vi "Checkout Master File.vi"(8 "error in":errorcluster, 10 "File Index":i32, 11 "Peer Review in":refnum<class "Peer Review.lvclass">) -> (0 "error out":errorcluster, 3 "Peer Review out":refnum<class "Peer Review.lvclass">)   [LabVIEW 2020, in "Peer Review.lvclass"]
uses:
  Peer Review.lvclass
  Peer Review.lvclass/Peer Review.ctl
  TypeDefs/File State.ctl
  <vilib>/security/Message Digest/API/Instances/File/SHA-256 File Checksum.vi
  <vilib>/security/Message Digest/API/NI_Message Digest API.lvlib
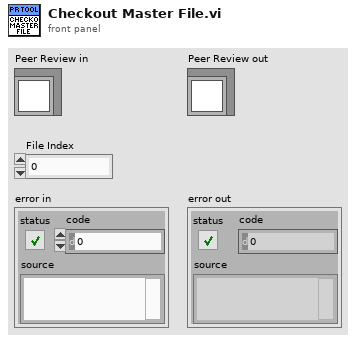
[diagram p1: front panel]
types:
  T1 = typedef "Peer Review.lvclass/File State.ctl" = enum16{"Interrogation Needed", "Modified", "Deleted", "Added", "Matches Previous", "No Changes", "Moved"}
  T2 = typedef "Peer Review.lvclass/File Info.ctl" = cluster{"File ID":i32, "Commit ID":i32, "Reviewed Hash":string, "Relative Path":string, "File Path":path, "File Checksum":string, "State":T1, "FP Changes":i32, "BD Changes":i32, "FP Bounds Error":dbl, "BD Bounds Error":dbl, "Lines Added":i32, "Lines Removed":i32, "Analysis Passes":i32, "Analysis Fails":i32, "Attribute Changes":i32, "Reentrancy State":string, "Cyclomatic Complexity":i32, "Node Count":i32, "Revision Number":u32, "LabVIEW Version":string, "Description":string, "Master Path":path, "Master Checksum":string, "VI Type":T3, "LabVIEW File":bool, "Review Complete":bool, "File Ref":refnum<vi>}
  T3 = typedef "Peer Review.lvclass/VI Type.ctl" = enum32{"invalid VI type", "Standard VI", "Control VI", "Global VI", "Polymorphic VI", "Configuration VI", "SubSystem", "Facade VI", "Method VI", "Statechart Diagram VI"}
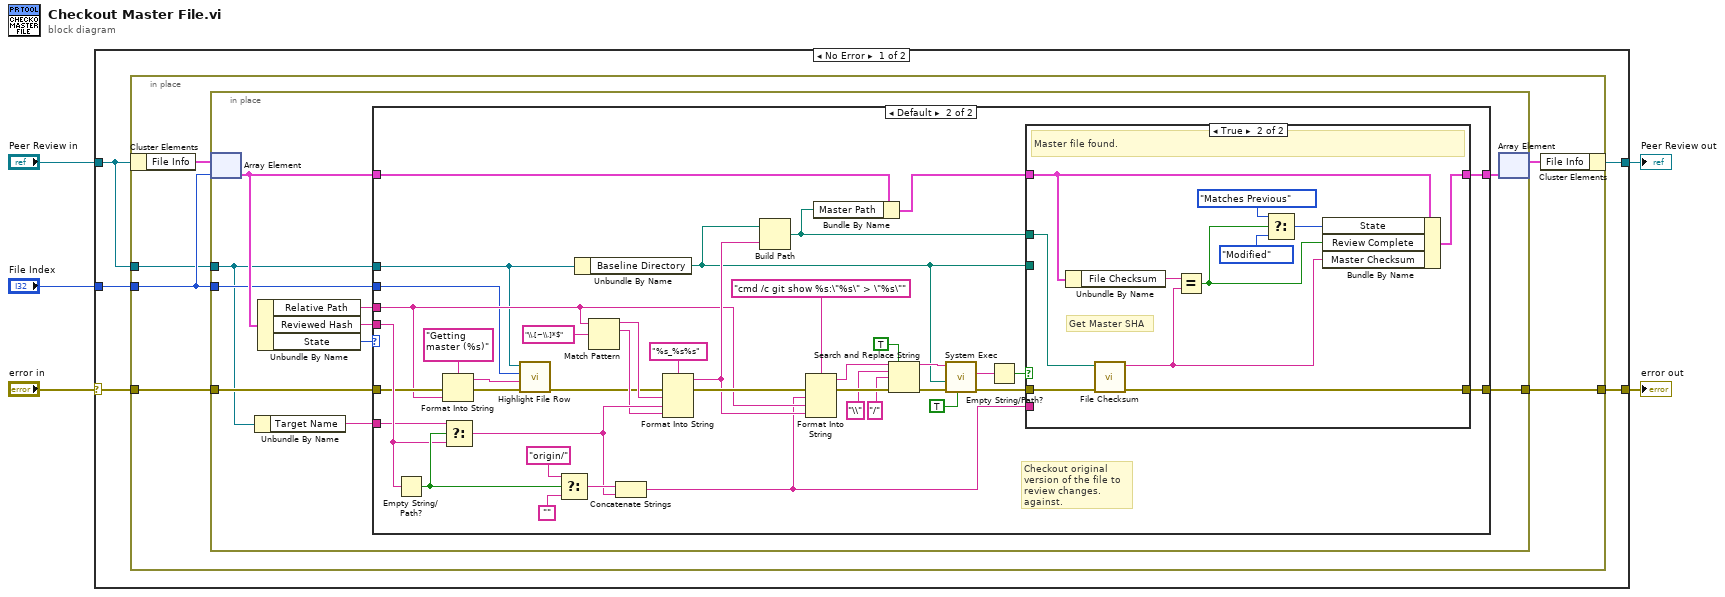
[diagram p0: block diagram]
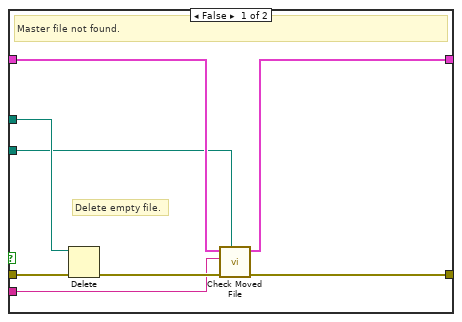
[diagram p3: hidden frame]
diagram:
  n1 = case shown="No Error" "error in" {
    selector: "error in" -> [w10 w89]
    tunnel: [w9 w89] -> w4
    tunnel: "Peer Review in" -> [w6 w88]
    tunnel: "File Index" -> [w8 _]
    tunnel: [w7 w88] -> w1
    frame No Error {
      n2 = in-place {
        in-place-border: w10 -> [w16]
        in-place-border: [w15] -> w9
        in-place-border: w8 -> [w12]
        in-place-border: w6 -> [w11]
        n3 = in-place-cluster #1(w6) -> ("File Info"=w14:T2[])
        n4 = in-place {
          in-place-border: w16 -> [w22]
          in-place-border: [w26] -> w15
          in-place-border: w12 -> [w20]
          in-place-border: w11 -> [w19]
          n5 = in-place-array #2(w14, w12) -> (w24:T2)
          n6 = Unbundle By Name(w19) -> ("Target Name"=w18:string)
          n7 = Unbundle By Name(w24) -> ("Relative Path"=w21:string, "Reviewed Hash"=w25:string, "State"=w17:T1)
          n8 = case shown="Default" w17 {
            tunnel: [w28 w57] -> w26
            tunnel: w25 -> [_ w42]
            tunnel: w24 -> [w27 w41]
            tunnel: [w27 w40] -> w23
            tunnel: w22 -> [w28 w35]
            tunnel: w21 -> [_ w34]
            tunnel: w20 -> [_ w33]
            tunnel: w19 -> [_ w30]
            tunnel: w18 -> [_ w29]
            frame "Deleted" {
            }
            frame Default {
              # "Checkout original version of the file to review changes. against."
              n9 = Empty String/Path?(string/path=w42) -> (empty?=w51:bool)
              n10 = Format Into String(format string="Getting master (%s)", error in=w35, w34) -> (resulting string=w38:string, error out=w39:errorcluster)  [unwired: 1 in]
              n11 = Select(t=w29, s=w51, f=w42) -> (s? t:f=w47:string)
              n12 = call "Highlight File Row.vi"("error in"=w39, "Status"=w38, "Current Row"=w33, "Peer Review"=w30) -> ("error out"=w36:errorcluster)  [unwired: 7 in]
              n13 = Select(t="origin/", s=w51, f="" ("Empty String Constant")) -> (s? t:f=w48:string)
              n14 = Unbundle By Name(w30) -> ("Baseline Directory"=w31:path)
              n15 = Match Pattern(string=w34, regular expression="\\.[~\\.]*$") -> (before substring=w65:string, match substring=w43:string)  [unwired: 3 out]
              n16 = Concatenate Strings(w48, w47) -> (w32:string)
              n17 = Format Into String(format string="%s_%s%s", error in=w36, w65, w47, w43) -> (resulting string=w64:string, error out=w66:errorcluster)  [unwired: 1 in]
              n18 = Build Path(base path=w31, name or relative path=w64) -> (appended path=w53:path)
              n19 = Format Into String(format string="cmd /c git show %s:\"%s\" > \"%s\"", error in=w66, w32, w34, w64) -> (resulting string=w63:string, error out=w62:errorcluster)  [unwired: 1 in]
              n20 = Bundle By Name(cluster=w41, "Master Path"=w53) -> (w55:T2)
              n21 = Search and Replace String(replace all?=TRUE ("replace all? (F)"), input string=w63, search string="\\", replace string="/", error in=w62) -> (result string=w52:string, error out=w61:errorcluster)  [unwired: 3 in, 2 out]
              n22 = call <vilib>:"System Exec.vi"("run minimized? (F)"=TRUE, "error in (no error)"=w61, "working directory"=w31, "command line"=w52) -> ("error out"=w56:errorcluster, "standard error"=w44:string)  [unwired: 4 in, 2 out]
              n23 = Empty String/Path?(string/path=w44) -> (empty?=w54:bool)
              n24 = case shown="True" w54 {
                tunnel: [w73 w78] -> w57
                tunnel: w56 -> [w76 w82]
                tunnel: w55 -> [w71 w81]
                tunnel: [w72 w80] -> w40
                tunnel: w53 -> [w75 w79]
                tunnel: w31 -> [w70 _]
                tunnel: w32 -> [w69 _]
                frame False {
                  # "Delete empty file."
                  # "Master file not found."
                  n25 = Delete(path (use dialog)=w75, error in=w76) -> (error out=w74:errorcluster)  [unwired: 3 in, 2 out]
                  n26 = call "Check Moved File.vi"("Baseline Directory"=w70, "error in"=w74, "Target"=w69, "File Info in"=w71) -> ("error out"=w73:errorcluster, "File Info out"=w72:T2)  [unwired: 6 in]
                }
                frame True {
                  # "Get Master SHA"
                  # "Master file found."
                  n27 = Unbundle By Name(w81) -> ("File Checksum"=w87:string)
                  n28 = call-poly <vilib>:"File Checksum.vi"("error in"=w82, "path"=w79) -> ("error out"=w78:errorcluster, "digest"=w77:string)  [unwired: 8 in]
                  n29 = Equal?(x=w87, y=w77) -> (x = y?=w83:bool)
                  n30 = Select(t=File_State."Matches Previous" ("File State"), s=w83, f=File_State."Modified" ("File State")) -> (s? t:f=w84:T1)
                  n31 = Bundle By Name(cluster=w81, "State"=w84, "Review Complete"=w83, "Master Checksum"=w77) -> (w80:T2)
                }
              }
            }
          }
          n32 = in-place-array #2(w23) -> (w13:T2[])  [unwired: 1 out]
        }
        n33 = in-place-cluster #1("File Info"=w13) -> (w7:refnum<class "Peer Review.lvclass">)
      }
    }
    frame Error {
    }
  }
  "error out" <- w4
  "Peer Review out" <- w1
